vi "Config hardware.vi"(8 "error in":errorcluster, 11 "Settings":T1={"Port"={"Port Name"="", "Board Type"=enum."Uno", "Baud Rate"=115200}, "Sample Rate (HZ)"=100, "Samples to Read"=50, "Input Pin"=0, "File path saved"=path ""}) -> (0 "error out":errorcluster, 3 "Settings out":T1={"Port"={"Port Name"="", "Board Type"=enum."Uno", "Baud Rate"=115200}, "Sample Rate (HZ)"=100, "Samples to Read"=50, "Input Pin"=0, "File path saved"=path ""})   [LabVIEW 2016]
uses:
  <vilib>/LabVIEW Interface for Arduino/Type Defs/Board Type.ctl
  Control/Settings.ctl
  Control/port config.ctl
  <vilib>/LabVIEW Interface for Arduino/LabVIEW Interface for Arduino.lvlib
panel:
  in  "Input Pin":u8
  in  "Cancel Button":bool
  in  "OK Button":bool
  in  "File name":string
  out "Boolean":bool caption="Configuration Arduino Board"
  in  "File Path":path
  in  "Samples to Read":u16=50
  in  "Sample Rate (HZ)":u16=100
  in  "Baud Rate":u32=115200
  in  "Board Type":T3
  in  "Port Name":refnum<visa-resource-name>
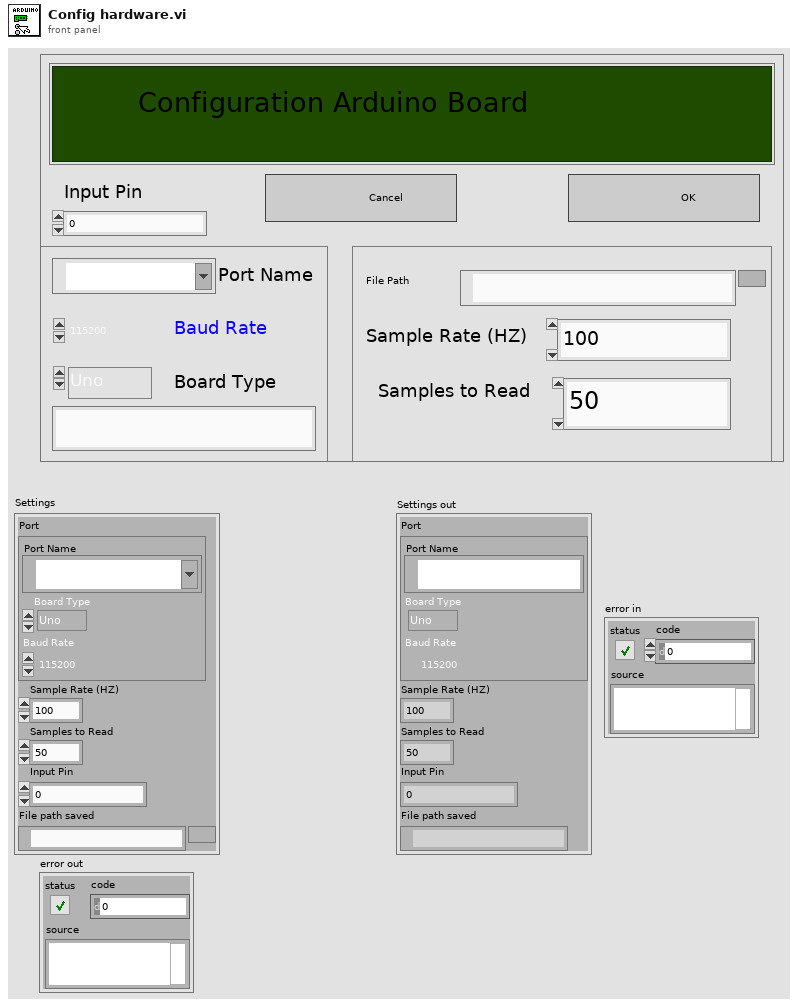
[diagram p1: front panel]
types:
  T1 = typedef "Settings.ctl" = cluster{"Port":T2, "Sample Rate (HZ)":u16, "Samples to Read":u16, "Input Pin":u8, "File path saved":path}
  T2 = typedef "port config.ctl" = cluster{"Port Name":refnum<visa-resource-name>, "Board Type":T3, "Baud Rate":u32}
  T3 = typedef "LabVIEW Interface for Arduino.lvlib/Board Type.ctl" = enum16{"Uno", "Dimuelanove w/Atmega 328", "Mega 2560"}
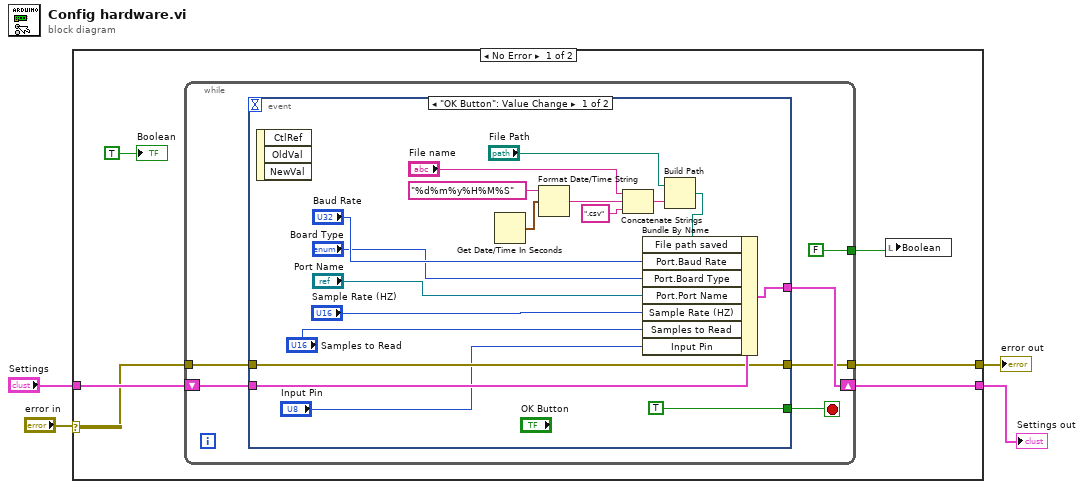
[diagram p0: block diagram]
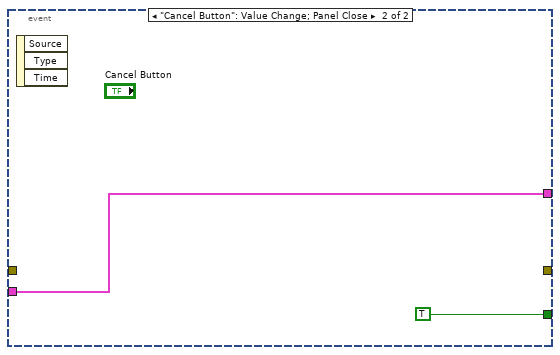
[diagram p2: hidden frame]
diagram:
  n1 = case shown="No Error" "error in" {
    selector: "error in" -> [w6 w37]
    tunnel: "Settings" -> [w10 w38]
    tunnel: [w8 w38] -> w2
    tunnel: [w5 w37] -> w1
    frame No Error {
      n2 = while {
        shift-right: [w14] -> w8
        shift-left: w10 -> [w15]
        tunnel: [FALSE] -> w7
        tunnel: w6 -> [w12]
        tunnel: [w11] -> w5
        stop <- w16 stop-if-true
        n3 = event shown="[0] \"OK Button\": Value Change" {
          selector: _ -> [_ _]
          dyn-events: _ -> [_ _]
          timeout: _ -> [_ _]
          tunnel: [TRUE TRUE] -> w16
          tunnel: w15 -> [w33 w35]
          tunnel: [w27 w35] -> w14
          tunnel: [w26 _] -> w11
          tunnel: w12 -> [w26 _]
          event "OK Button": Value Change {
            n4 = event-data() -> ()  [unwired: 1 in, 3 out]
            n5 = Get Date/Time In Seconds() -> (seconds since 1Jan1904=w23:timestamp)
            n6 = Format Date/Time String(time format string (%c)="%d%m%y%H%M%S", seconds (now)=w23) -> (date/time string=w24:string)  [unwired: 1 in]
            n7 = Concatenate Strings("File name", w24, ".csv") -> (w22:string)
            n8 = Build Path(base path="File Path", name or relative path=w22) -> (appended path=w17:path)
            n9 = Bundle By Name(cluster=w33, "File path saved"=w17, "Port.Baud Rate"="Baud Rate", "Port.Board Type"="Board Type", "Port.Port Name"="Port Name", "Sample Rate (HZ)"="Sample Rate (HZ)", "Samples to Read"="Samples to Read", "Input Pin"="Input Pin") -> (w27:T1)
          }
          event "Cancel Button": Value Change; Panel Close {
            n10 = event-data() -> ()  [unwired: 1 in, 3 out]
          }
        }
      }
      n11 = local write "Boolean"(w7) -> ()
      "Boolean" <- TRUE ("Boolean")
    }
    frame Error {
    }
  }
  "Settings out" <- w2
  "error out" <- w1
